vi "test 02.vi"() -> ()   [LabVIEW 2020]
uses:
  UI_Actor/UI_Actor/UI_Actor.lvclass
panel:
  in  "Path":path
  in  "String":string
  in  "Boolean":bool
  in  "Numeric":dbl
  in  "Cluster":T1
  out "PASS":bool
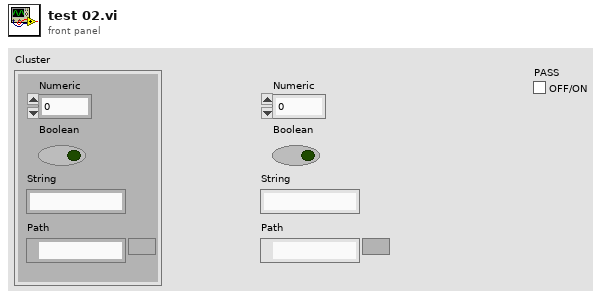
[diagram p1: front panel]
types:
  T1 = cluster{"Numeric":dbl, "Boolean":bool, "String":string, "Path":path}
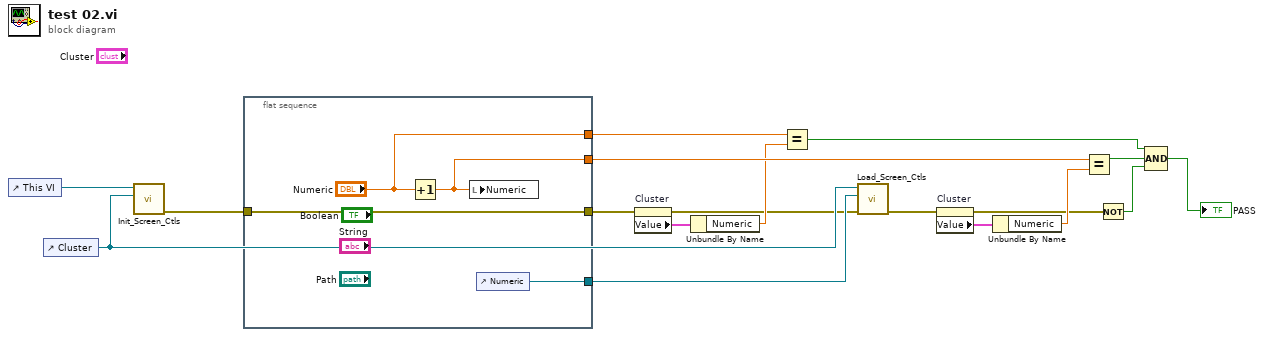
[diagram p0: block diagram]
diagram:
  n1 = control-ref of="This VI"() -> (w18:refnum<vi>)
  n2 = control-ref of="Cluster"() -> (w17:refnum<vi>)
  n3 = call "Init_Screen_Ctls.vi"("Cluster to load"=w17, "VI ref"=w18) -> ("error out"=w16:errorcluster)  [unwired: 7 in, 2 out]
  n4 = flat-sequence {
    tunnel: [w22] -> w8
    tunnel: w16 -> [w22]
    tunnel: [w21] -> w15
    tunnel: [w20] -> w12
    tunnel: ["Numeric"] -> w7
    frame #0 {
      n5 = Increment(x="Numeric") -> (x+1=w20:dbl)
      n6 = local write "Numeric"(w20) -> ()
      n7 = control-ref of="Numeric"() -> (w21:refnum<vi>)
    }
  }
  n8 = property on="Cluster" class="Clust (strict)"(error in=w8) -> (error out=w6:errorcluster, "Value"=w9:T1)  [unwired: 1 in, 1 out]
  n9 = Unbundle By Name(w9) -> ("Numeric"=w10:dbl)
  n10 = Equal?(x=w7, y=w10) -> (x = y?=w5:bool)
  n11 = call "Load_Screen_Ctls.vi"("error out"=w6, "CtlRef"=w15, "Cluster to change"=w17) -> ("error out"=w14:errorcluster)  [unwired: 7 in, 1 out]
  n12 = property on="Cluster" class="Clust (strict)"(error in=w14) -> (error out=w3:errorcluster, "Value"=w13:T1)  [unwired: 1 in, 1 out]
  n13 = Unbundle By Name(w13) -> ("Numeric"=w11:dbl)
  n14 = Equal?(x=w12, y=w11) -> (x = y?=w4:bool)
  n15 = Not(x=w3) -> (.not. x?=w2:bool)
  n16 = Compound Arithmetic op=AND(w5, w4, w2) -> (→"PASS":bool)
